vi "DG convert (SubVI).vi"(4 "String":string, 5 "Reset pressure":bool, 6 "atm kPa":dbl=10.0, 7 "manual reset":bool) -> (0 "depth":dbl=100000.0 format="%#.1f", 1 "UNI depth":dbl, 3 "Pressure (deciBAR = 10*kPASCAL)":dbl=100000.0 format="%#.1f")   [LabVIEW 2014]
uses:
  Helping Routines/get_set_point (SubVI).vi
  <vilib>/imath/engines/lvmath2/RunTimeEngine/NodeEndStatement/NIMS_NodeEndStatement_Output.vi
  <instcachedir>/0/NIMS_NodeEndStatement_Output_53EC0D466D134D7ABD903AC30B43404B.lvgen/NIMS_NodeEndStatement_Output_53EC0D466D134D7ABD903AC30B43404B_001.vi
  <vilib>/imath/engines/lvmath2/RunTimeEngine/ErrorHandling/NIMS_Finalize Error.vi
panel:
  in  "UNI depth ON":bool=TRUE
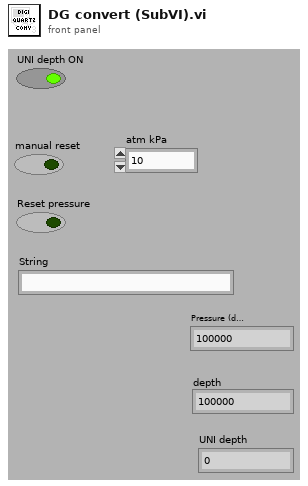
[diagram p1: front panel]
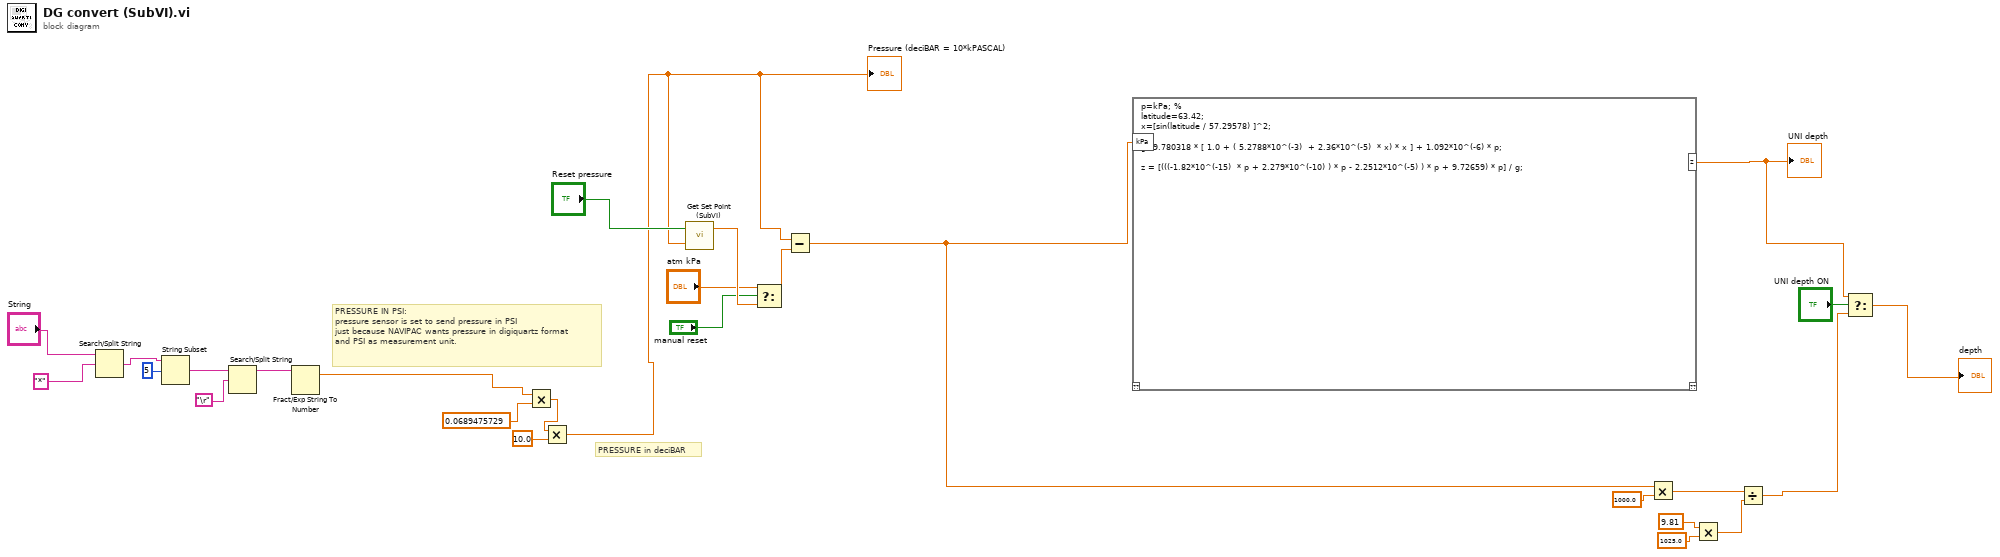
[diagram p0: block diagram]
diagram:
  # "PRESSURE in deciBAR"
  # "PRESSURE IN PSI:\npressure sensor is set to send pressure in PSI\njust because NAVIPAC wants pressure in digiquartz format and PSI as measurement unit."
  n1 = Search/Split String(string="String", search string/char (-)="*") -> (match + rest of string=w23:string)  [unwired: 1 in, 2 out]
  n2 = String Subset(string=w23, offset (0)=5) -> (substring=w22:string)  [unwired: 1 in]
  n3 = Search/Split String(string=w22, search string/char (-)="\r") -> (substring before match=w21:string)  [unwired: 1 in, 2 out]
  n4 = Fract/Exp String To Number(string=w21) -> (number=w3:dbl)  [unwired: 3 in, 1 out]
  n5 = Multiply(x=w3, y=0.0689475729) -> (x*y=w5:dbl)
  n6 = Multiply(x=w5, y=10.0) -> (x*y=w2:dbl)
  "Pressure (deciBAR = 10*kPASCAL)" <- w2
  n7 = call-poly "Get Set Point (SubVI).vi"("set point in"=w2, "auto set  in"="Reset pressure") -> ("set point"=w14:dbl)  [unwired: 1 out]
  n8 = Select(t="atm kPa", s="manual reset", f=w14) -> (s? t:f=w13:dbl)
  n9 = Subtract(x=w2, y=w13) -> (x-y=w10:dbl)
  n10 = mathscript code="p=kPa; %\nlatitude=63.42;\nx=[sin(latitude / 57.29578) ]^2;\n\ng=9.780318 * [ 1.0 + ( 5.2788*10^(-3)  + 2.36*10^(-5)  * x) * x ] + 1.092*10^(-6) * p;\n\nz = [(((-1.82*10^(-15)  * p + 2.279*10^(-10) ) * p - 2.2512*10^(-5) ) * p + 9.72659) * p] / g;"("kPa"=w10) -> ("z"=w8:dbl)  [unwired: 1 in, 1 out]
  "UNI depth" <- w8
  n11 = Multiply(x=w10, y=1000.0) -> (x*y=w17:dbl)
  n12 = Multiply(x=9.81, y=1025.0) -> (x*y=w16:dbl)
  n13 = Divide(x=w17, y=w16) -> (x/y=w7:dbl)
  n14 = Select(t=w8, s="UNI depth ON", f=w7) -> (s? t:f=→"depth":dbl)
